vi "面罩Debug.vi"() -> ()   [LabVIEW 2015]
uses:
  <vilib>/Platform/TimedLoop/XDataNode/timing_clust.ctl
  <vilib>/Platform/TimedLoop/XDataNode/nitl_modes.ctl
  <vilib>/Platform/TimedLoop/XDataNode/wakeup.ctl
  <vilib>/Instr/_visa.llb/VISA Configure Serial Port (Instr).vi
  <vilib>/Platform/TimedLoop/XDataNode/XDataNode.xnode
  <vilib>/Platform/TimedLoop/XDataNode/XDNodeRunTimeDep.lvlib
panel:
  in  "HEX发送":bool
  in  "组合框Combox":T1
  in  "十六进制发送":bool
  in  "十六进制 Text":string
  in  "字符串按钮":bool
  in  "字符串 Text":string
  out "写入历史":string
  in  "写入缓冲区":string
  out "错误输出":errorcluster
  in  "发送控制协议":bool
  in  "速度":u16(slide) scale=0.0..100.0
  in  "位置":u16(slide) scale=0.0..90.0
  in  "清空":bool
  in  "停止":bool
  in  "暂停/恢复":bool
  out "读取缓冲区":string
  out "返回数":u32
  in  "baud rate (115200)":u32=115200 caption="波特率(115200)"
  in  "VISA resource name":refnum<visa-resource-name> caption="串口"
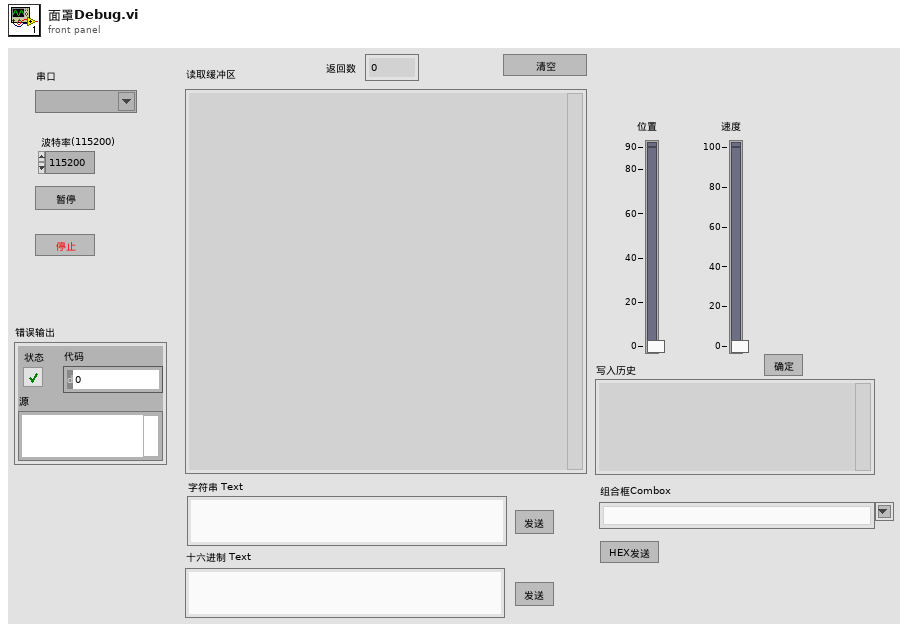
[diagram p1: front panel]
types:
  T1 = typedef "控件 1.ctl" = string
  T2 = typedef "XDNodeRunTimeDep.lvlib/timing_clust.ctl" = cluster{"Expected End [f-1]":u64, "Actual End [f-1]":u64, "Finished Late? [f-1]":bool, "Expected End [i-1]":u64, "Actual End [i-1]":u64, "Finished Late? [i-1]":bool, "Expected Start [i]":u64, "Actual Start [i]":u64, "Expected Start [f]":u64, "Actual Start [f]":u64, "Source Name":string, "Structure Name":string, "Period":i64, "Deadline":i64, "Offset":i64, "Start":i64, "Priority":i32, "Timeout":i32, "Mode":T3, "Wakeup Reason":T4, "Error":errorcluster, "Source Type":string, "Secondary Source Type":string, "Global End Time":u64, "Global Start Time":u64, "Frame Duration":u64, "Iteration Duration":u64, "Assigned CPU":i32, "I/O Scan Engine Mode":u32}
  T3 = typedef "XDNodeRunTimeDep.lvlib/nitl_modes.ctl" = enum32{"No Change", "Process missed periods, maintain original phase", "Discard missed periods, maintain original phase", "Process missed periods, ignore original phase", "Discard missed periods, ignore original phase"}
  T4 = typedef "XDNodeRunTimeDep.lvlib/wakeup.ctl" = enum32{"Normal", "Aborted", "Asynchronous wakeup", "Timing source error", "Timed loop error", "Timeout"}
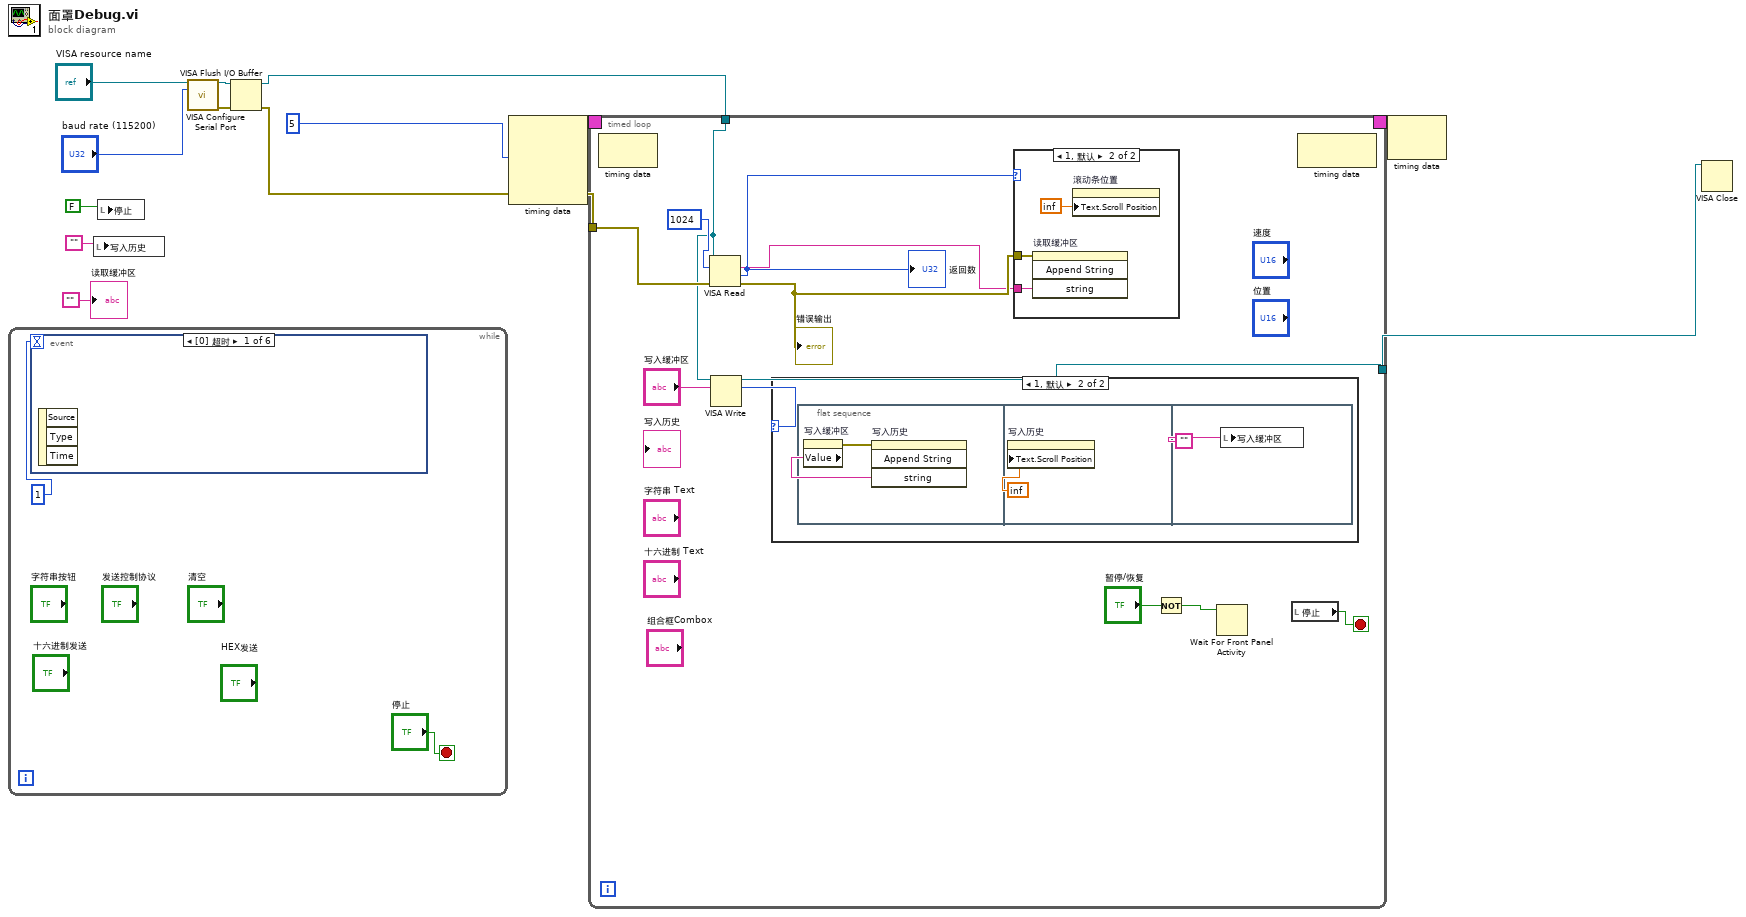
[diagram p0: block diagram]
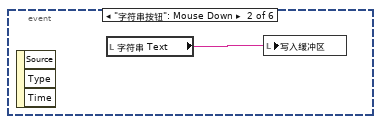
[diagram p2: hidden frame]
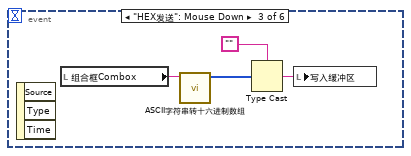
[diagram p3: hidden frame]
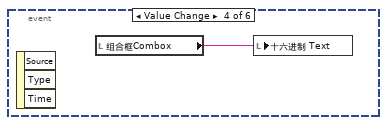
[diagram p4: hidden frame]
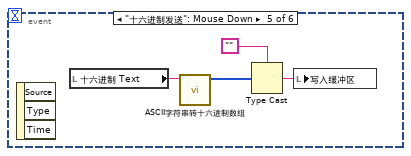
[diagram p5: hidden frame]
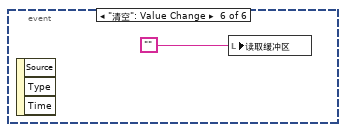
[diagram p6: hidden frame]
diagram:
  n1 = while {
    stop <- "停止" stop-if-true
    n2 = event shown="[0] 超时" {
      selector: _ -> [_ _ _ _ _ _]
      dyn-events: _ -> [_ _ _ _ _ _]
      timeout: 1 -> [_ _ _ _ _ _]
      event Timeout {
        n3 = event-data() -> ()  [unwired: 1 in, 3 out]
      }
      event "字符串按钮": Mouse Down {
        n4 = event-data() -> ()  [unwired: 1 in, 3 out]
        n5 = local read "字符串 Text"() -> (w16:string)
        n6 = local write "写入缓冲区"(w16) -> ()
      }
      event "HEX发送": Mouse Down {
        n7 = event-data() -> ()  [unwired: 1 in, 3 out]
        n8 = local read "组合框Combox"() -> (w20:T1)
        n9 = call "ASCII字符串转十六进制数组.vi"("字符"=w20) -> ("数组"=w18:u8[])  [unwired: 10 in]
        n10 = Type Cast(type="", x=w18) -> (*(type *) &x=w17:string)
        n11 = local write "写入缓冲区"(w17) -> ()
      }
      event Value Change {
        n12 = event-data() -> ()  [unwired: 1 in, 3 out]
        n13 = local read "组合框Combox"() -> (w21:T1)
        n14 = local write "十六进制 Text"(w21) -> ()
      }
      event "十六进制发送": Mouse Down {
        n15 = event-data() -> ()  [unwired: 1 in, 3 out]
        n16 = local read "十六进制 Text"() -> (w25:string)
        n17 = call "ASCII字符串转十六进制数组.vi"("字符"=w25) -> ("数组"=w23:u8[])  [unwired: 10 in]
        n18 = Type Cast(type="", x=w23) -> (*(type *) &x=w22:string)
        n19 = local write "写入缓冲区"(w22) -> ()
      }
      event "清空": Value Change {
        n20 = event-data() -> ()  [unwired: 1 in, 3 out]
        n21 = local write "读取缓冲区"("") -> ()
      }
    }
  }
  n22 = local write "写入历史"("") -> ()
  n23 = local write "停止"(FALSE) -> ()
  n24 = call-poly "VISA Configure Serial Port"("VISA resource name"="VISA resource name", "baud rate (9600)"="baud rate (115200)") -> ("VISA resource name out"=w7:refnum<visa-resource-name>, "error out"=w6:errorcluster)  [unwired: 12 in]
  n25 = VISA Flush I/O Buffer(VISA resource name=w7, error in (no error)=w6) -> (VISA resource name out=w8:refnum<visa-resource-name>, error out=w5:errorcluster)  [unwired: 1 in]
  n26 = node-c288(i64 5 ("周期")) -> (w11:T2)  [unwired: 3 in]
  n27 = timed-loop {
    tunnel: w8 -> [w28]
    timing: w11 -> [_]
    timing-out: [_] -> w10
    tunnel: w5 -> [w36]
    tunnel: [w30] -> w3
    stop <- w27 stop-if-true
    n28 = node-c288() -> ()  [unwired: 1 in, 1 out]
    n29 = VISA Read(VISA resource name=w28, byte count=u32 1024 ("字节总数"), error in (no error)=w36) -> (read buffer=w37:string, return count=w34:u32, error out=w38:errorcluster)  [unwired: 1 out]
    "返回数" <- w34
    "错误输出" <- w38
    n30 = VISA Write(VISA resource name=w28, write buffer="写入缓冲区") -> (VISA resource name out=w30:refnum<visa-resource-name>, return count=w29:u32)  [unwired: 1 in, 1 out]
    n31 = case shown="1, 默认" w29 {
      frame 0 {
      }
      frame 1, Default {
        n32 = flat-sequence {
          frame #0 {
            n33 = property on="写入缓冲区" class="Str"() -> (error out=w39:errorcluster, "Value"=w40:string)  [unwired: 2 in, 1 out]
            n34 = invoke on="写入历史" class="Str" method="Append String"(error in=w39, "string"=w40) -> ()  [unwired: 2 in, 4 out]
          }
          frame #1 {
            n35 = property on="写入历史" class="Str"("Text.Scroll Position"=inf) -> ()  [unwired: 2 in, 2 out]
          }
          frame #2 {
            n36 = local write "写入缓冲区"("") -> ()
          }
        }
      }
    }
    n37 = case shown="1, 默认" w34 {
      tunnel: w37 -> [_ w47]
      tunnel: w38 -> [_ w46]
      frame 0 {
      }
      frame 1, Default {
        n38 = invoke on="读取缓冲区" class="Str" method="Append String"(error in=w46, "string"=w47) -> ()  [unwired: 2 in, 4 out]
        n39 = property on="滚动条位置" class="Str"("Text.Scroll Position"=inf) -> ()  [unwired: 2 in, 2 out]
      }
    }
    n40 = Not(x="暂停/恢复") -> (.not. x?=w32:bool)
    n41 = Wait For Front Panel Activity(3:w32) -> ()  [unwired: 2 in, 1 out]
    n42 = local read "停止"() -> (w27:bool)
    n43 = node-c288() -> ()  [unwired: 1 in, 1 out]
  }
  n44 = node-c288(w10) -> ()  [unwired: 1 out]
  n45 = VISA Close(VISA resource name=w3) -> ()  [unwired: 1 in, 1 out]
  "读取缓冲区" <- ""
